vi "PSAE_VCH_Update Data Structure.vi"(8 "Error In (no error)":errorcluster, 10 "Call Data":variant, 11 "Popup Value":variant) -> (0 "Error Out":errorcluster, 3 "Giveup？":bool)   [LabVIEW 2016]
uses:
  <vilib>/Pansino Software/ToolkitLib/Popup Toolkit/Private/Ctrls/PSPOP_Grid.Cell Info.ctl
  <vilib>/Pansino Software/ToolkitLib/Popup Toolkit/Private/Ctrls/PSPOP_Data Type.ctl
panel:
  # "Data Out"
  # "Data In"
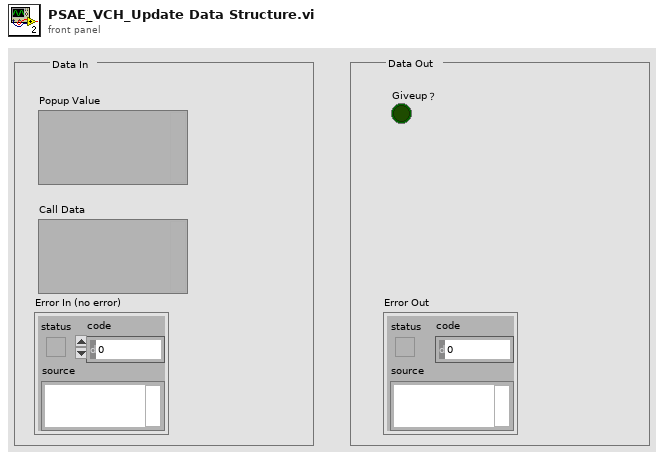
[diagram p1: front panel]
types:
  T1 = typedef "PSPOP_Grid.Cell Info.ctl" = cluster{"Tag":string, "Row":i32, "Column":i32, "In Symbol?":bool, "In Data?":bool, "Cell String":string, "Ctl Refnum":refnum<vi>, "Prop Type":T2, "Ring Strings":string[], "Ring Values":ext[], "New Cell String":string}
  T2 = typedef "PSPOP_Data Type.ctl" = enum16{"NO POPUP", "Unkown", "String", "Integer", "Float", "Color", "Boolean", "Ring", "Captioned String", "Captioned Integer", "Button Color", "2 Int Cluster", "4 Int Cluster", "6-Dbl Cluster", "Path", "Combox", "Time", "ShotCut String"}
  T3 = typedef "PSVCH_VCH Info.ctl" = cluster{"Tag":string[], "Tag String":string[], "Name":string[], "Enable":bool[], "Formula":string[], "Unit":string[], "Save":bool[], "Time":i64[]}
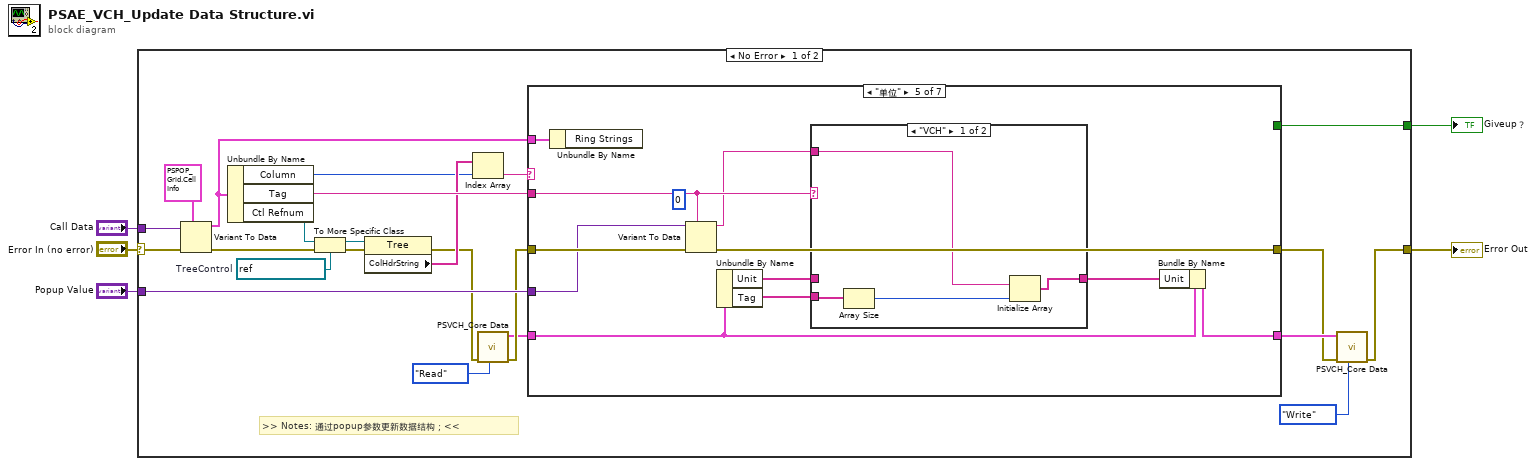
[diagram p0: block diagram]
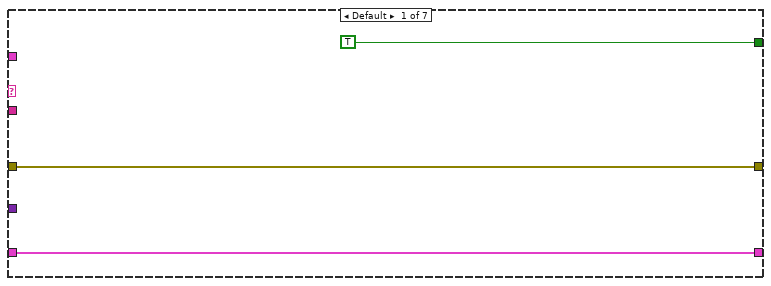
[diagram p2: hidden frame]
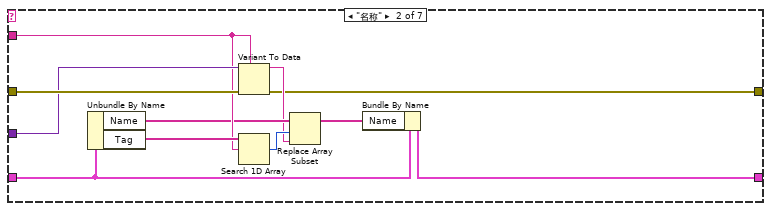
[diagram p3: hidden frame]
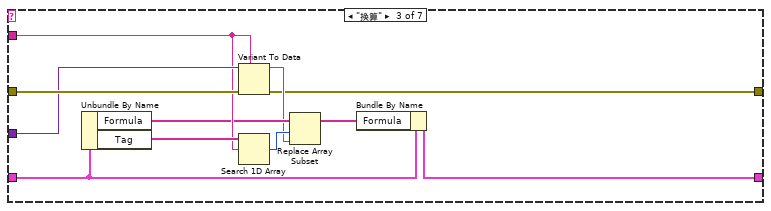
[diagram p4: hidden frame]
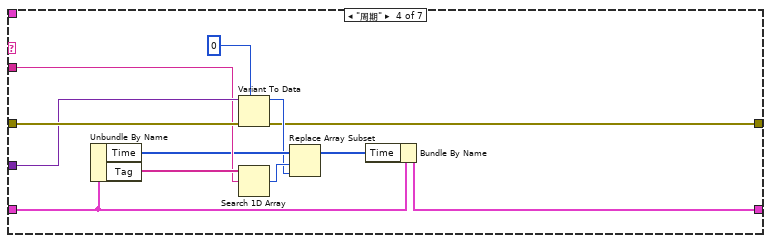
[diagram p5: hidden frame]
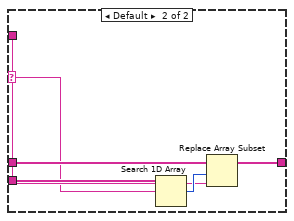
[diagram p6: hidden frame]
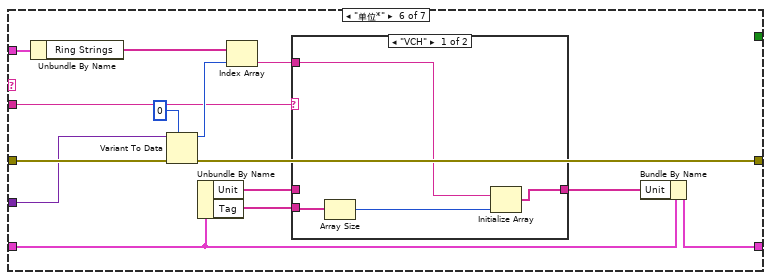
[diagram p7: hidden frame]
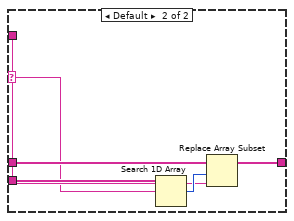
[diagram p8: hidden frame]
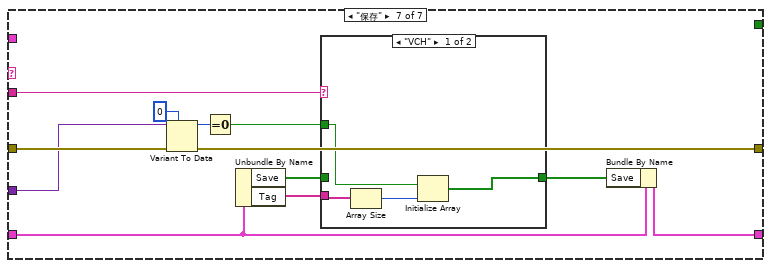
[diagram p9: hidden frame]
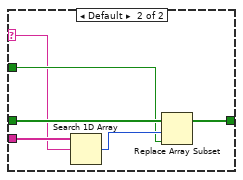
[diagram p10: hidden frame]
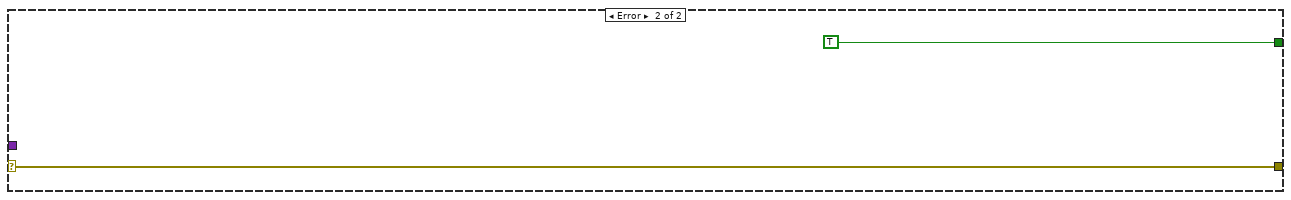
[diagram p11: hidden frame]
diagram:
  n1 = case shown="No Error" "Error In (no error)" {
    selector: "Error In (no error)" -> [w16 w134]
    tunnel: "Popup Value" -> [w27 _]
    tunnel: "Call Data" -> [w22 _]
    tunnel: [w8 w134] -> w3
    tunnel: [w14 TRUE] -> w1
    frame No Error {
      w20 = refnum<vi> refnum  # TreeControl
      # ">> Notes: 通过popup参数更新数据结构；<<"
      n2 = Variant To Data(error in=w16, type=T1 {"Tag"="", "Row"=0, "Column"=0, "In Symbol?"=FALSE, "In Data?"=FALSE, "Cell String"="", "Ctl Refnum"=refnum, "Prop Type"=enum."Unkown", "Ring Strings"=[], "Ring Values"=[], "New Cell String"=""} ("Cell Info (type only)"), Variant=w22) -> (data=w15:T1, error out=w19:errorcluster)
      n3 = Unbundle By Name(w15) -> ("Column"=w24:i32, "Tag"=w28:string, "Ctl Refnum"=w21:refnum<vi>)
      n4 = To More Specific Class(target class=w20, reference=w21, error in=w19) -> (specific class reference=w17:refnum<vi>, error out=w18:errorcluster)
      n5 = property class="Tree"(reference=w17, error in=w18) -> (error out=w13:errorcluster, "ColHdrString"=w25:string[])  [unwired: 1 out]
      n6 = Index Array(array=w25, index=w24) -> (element=w26:string)
      n7 = call "PSVCH_Core Data.vi"("Oper"=enum16{"Init", "Read", "Write"}."Read", "Error In (no error)"=w13) -> ("Error Out"=w12:errorcluster, "VCH Out"=w11:T3)  [unwired: 8 in]
      n8 = case shown="\"单位\"" w26 {
        tunnel: w11 -> [w30 w34 w45 w57 w71 w95 w117]
        tunnel: w12 -> [w31 w42 w53 w65 w76 w100 w122]
        tunnel: [w31 w35 w46 w58 w72 w96 w118] -> w9
        tunnel: [w30 w32 w43 w55 w69 w93 w115] -> w10
        tunnel: w27 -> [_ w41 w52 w64 w75 w99 w121]
        tunnel: w28 -> [_ w39 w50 w62 w67 w87 w111]
        tunnel: w15 -> [_ _ _ _ w68 w92 _]
        tunnel: [TRUE _ _ _ _ _ _] -> w14
        frame Default {
        }
        frame "名称" {
          n9 = Unbundle By Name(w34) -> ("Name"=w38:string[], "Tag"=w40:string[])
          n10 = Variant To Data(error in=w42, type=w39, Variant=w41) -> (data=w36:string, error out=w35:errorcluster)
          n11 = Search 1D Array(1D array=w40, element=w39) -> (index of element=w37:i32)  [unwired: 1 in]
          n12 = Replace Array Subset(array=w38, new element=w36, index=w37) -> (w33:string[])
          n13 = Bundle By Name(cluster=w34, "Name"=w33) -> (w32:T3)
        }
        frame "换算" {
          n14 = Unbundle By Name(w45) -> ("Formula"=w49:string[], "Tag"=w51:string[])
          n15 = Variant To Data(error in=w53, type=w50, Variant=w52) -> (data=w47:string, error out=w46:errorcluster)
          n16 = Search 1D Array(1D array=w51, element=w50) -> (index of element=w48:i32)  [unwired: 1 in]
          n17 = Replace Array Subset(array=w49, new element=w47, index=w48) -> (w44:string[])
          n18 = Bundle By Name(cluster=w45, "Formula"=w44) -> (w43:T3)
        }
        frame "周期" {
          n19 = Unbundle By Name(w57) -> ("Time"=w61:i64[], "Tag"=w63:string[])
          n20 = Variant To Data(error in=w65, type=i64 0, Variant=w64) -> (data=w59:i64, error out=w58:errorcluster)
          n21 = Search 1D Array(1D array=w63, element=w62) -> (index of element=w60:i32)  [unwired: 1 in]
          n22 = Replace Array Subset(array=w61, new element=w59, index=w60) -> (w56:i64[])
          n23 = Bundle By Name(cluster=w57, "Time"=w56) -> (w55:T3)
        }
        frame "单位" {
          (unwired) 0
          n24 = Unbundle By Name(w68) -> ()  [unwired: 1 out]
          n25 = Variant To Data(error in=w76, type=w67, Variant=w75) -> (data=w66:string, error out=w72:errorcluster)
          n26 = Unbundle By Name(w71) -> ("Unit"=w73:string[], "Tag"=w74:string[])
          n27 = case shown="\"VCH\"" w67 {
            selector: w67 -> [_ w81]
            tunnel: w74 -> [w80 w86]
            tunnel: w73 -> [_ w85]
            tunnel: [w77 w83] -> w70
            tunnel: w66 -> [w79 w82]
            frame "VCH" {
              n28 = Array Size(array=w80) -> (size(s)=w78:i32)
              n29 = Initialize Array(w79, w78) -> (w77:string[])
            }
            frame Default {
              n30 = Search 1D Array(1D array=w86, element=w81) -> (index of element=w84:i32)  [unwired: 1 in]
              n31 = Replace Array Subset(array=w85, new element=w82, index=w84) -> (w83:string[])
            }
          }
          n32 = Bundle By Name(cluster=w71, "Unit"=w70) -> (w69:T3)
        }
        frame "单位*" {
          n33 = Unbundle By Name(w92) -> ("Ring Strings"=w90:string[])
          n34 = Variant To Data(error in=w100, type=0, Variant=w99) -> (data=w89:i32, error out=w96:errorcluster)
          n35 = Unbundle By Name(w95) -> ("Unit"=w97:string[], "Tag"=w98:string[])
          n36 = Index Array(array=w90, index=w89) -> (element=w88:string)
          n37 = case shown="\"VCH\"" w87 {
            selector: w87 -> [_ w105]
            tunnel: w98 -> [w104 w110]
            tunnel: w97 -> [_ w109]
            tunnel: [w101 w107] -> w94
            tunnel: w88 -> [w103 w106]
            frame "VCH" {
              n38 = Array Size(array=w104) -> (size(s)=w102:i32)
              n39 = Initialize Array(w103, w102) -> (w101:string[])
            }
            frame Default {
              n40 = Search 1D Array(1D array=w110, element=w105) -> (index of element=w108:i32)  [unwired: 1 in]
              n41 = Replace Array Subset(array=w109, new element=w106, index=w108) -> (w107:string[])
            }
          }
          n42 = Bundle By Name(cluster=w95, "Unit"=w94) -> (w93:T3)
        }
        frame "保存" {
          n43 = Variant To Data(error in=w122, type=0, Variant=w121) -> (data=w113:i32, error out=w118:errorcluster)
          n44 = Equal To 0?(x=w113) -> (x = 0?=w112:bool)
          n45 = Unbundle By Name(w117) -> ("Save"=w119:bool[], "Tag"=w120:string[])
          n46 = case shown="\"VCH\"" w111 {
            selector: w111 -> [_ w127]
            tunnel: w120 -> [w126 w132]
            tunnel: w119 -> [_ w131]
            tunnel: [w123 w129] -> w116
            tunnel: w112 -> [w124 w128]
            frame "VCH" {
              n47 = Array Size(array=w126) -> (size(s)=w125:i32)
              n48 = Initialize Array(w124, w125) -> (w123:bool[])
            }
            frame Default {
              n49 = Search 1D Array(1D array=w132, element=w127) -> (index of element=w130:i32)  [unwired: 1 in]
              n50 = Replace Array Subset(array=w131, new element=w128, index=w130) -> (w129:bool[])
            }
          }
          n51 = Bundle By Name(cluster=w117, "Save"=w116) -> (w115:T3)
        }
      }
      n52 = call "PSVCH_Core Data.vi"("Oper"=enum16{"Init", "Read", "Write"}."Write", "Error In (no error)"=w9, "VCH In"=w10) -> ("Error Out"=w8:errorcluster)  [unwired: 7 in, 1 out]
    }
    frame Error {
    }
  }
  "Error Out" <- w3
  "Giveup？" <- w1
